vi "aoc-2025-d01-2.vi"() -> ()   [LabVIEW 2020]
uses:
  <vilib>/Utility/miscctls.llb/LVRowAndColumnTypeDef.ctl
panel:
  out "min value":i32
  out "max value":i32
  out "Table Control":string[][](table)
  out "answer":i32
  out "input":i32[](array[numeric])
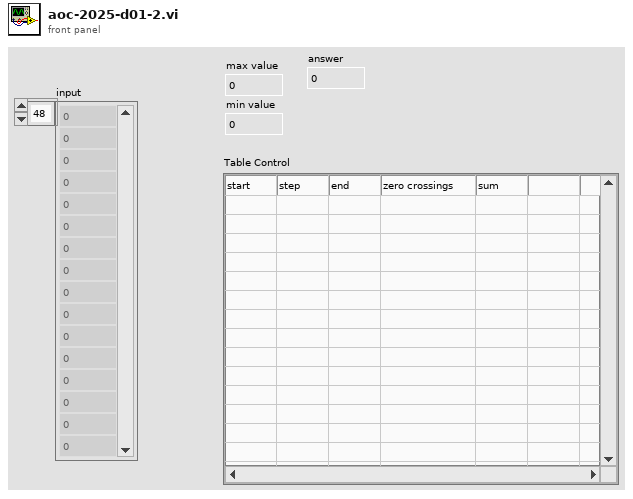
[diagram p1: front panel]
types:
  T1 = typedef "LVRowAndColumnTypeDef.ctl" = cluster{"Row":i32, "Column":i32}
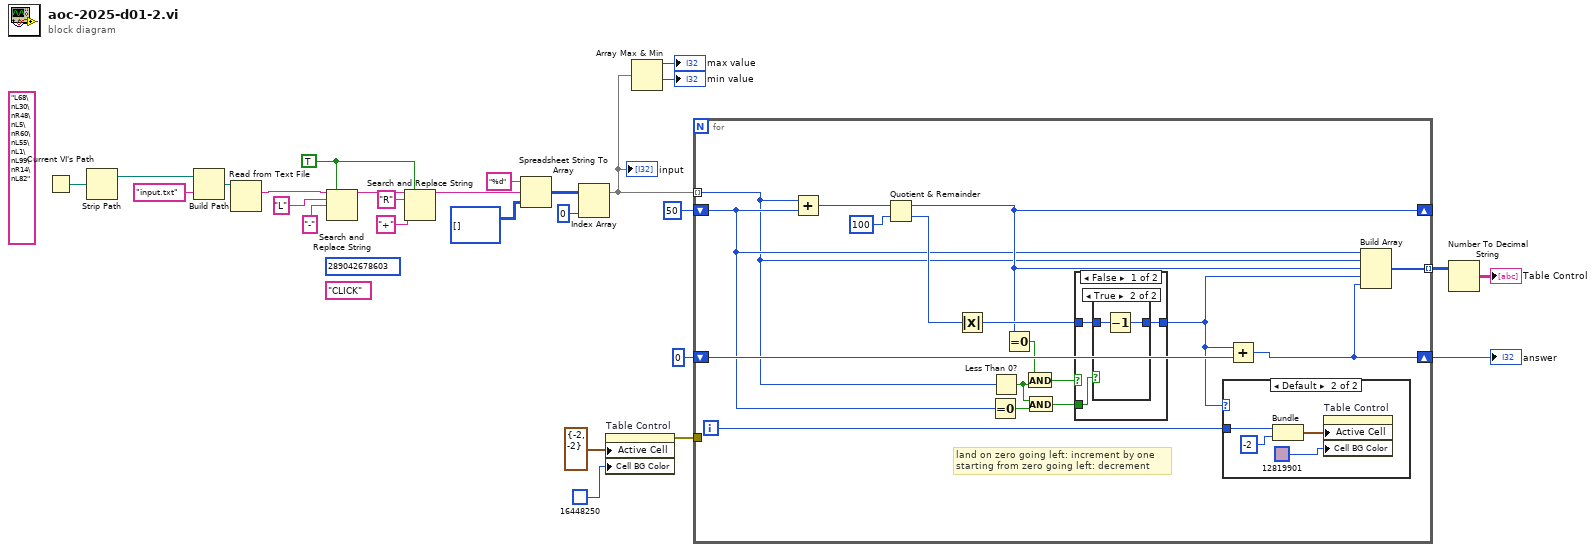
[diagram p0: block diagram]
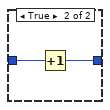
[diagram p3: hidden frame]
diagram:
  (unwired) "CLICK"
  (unwired) u64 289042678603
  (unwired) "L68\nL30\nR48\nL5\nR60\nL55\nL1\nL99\nR14\nL82"
  w26 = TRUE ("replace all? (F)")
  n1 = Current VI's Path() -> (path=w17:path)
  n2 = Strip Path(path=w17) -> (stripped path=w16:path)  [unwired: 1 out]
  n3 = Build Path(base path=w16, name or relative path="input.txt") -> (appended path=w14:path)
  n4 = Read from Text File(file (use dialog)=w14) -> (text=w8:string)  [unwired: 3 in, 3 out]
  n5 = Search and Replace String(replace all?=w26, input string=w8, search string="L" ("replace string (\"\")"), replace string="-" ("replace string (\"\")")) -> (result string=w27:string)  [unwired: 4 in, 3 out]
  n6 = Search and Replace String(replace all?=w26, input string=w27, search string="R", replace string="+" ("replace string (\"\")")) -> (result string=w9:string)  [unwired: 4 in, 3 out]
  n7 = Spreadsheet String To Array(format string="%d", spreadsheet string=w9, array type (2D Dbl)=i32[][] []) -> (array=w7:i32[][])  [unwired: 1 in]
  n8 = Index Array(array=w7, index (col)=0 ("disabled index (col)")) -> (element=w6:i32[])  [unwired: 1 in]
  "input" <- w6
  n9 = property on="Table Control" class="Tbl (strict)"("Active Cell"=T1 {"Row"=-2, "Column"=-2} ("Active Cell:Active Cell"), "Cell BG Color"=u32 16448250 ("Active Cell:Cell Background Color")) -> (error out=w3:errorcluster)  [unwired: 2 in, 1 out]
  n10 = Array Max & Min(array=w6) -> (max value=→"max value":i32, min value=→"min value":i32)  [unwired: 2 out]
  n11 = for {
    tunnel: w6 -> [w28] mode=indexing
    shift-right: [w34] -> _
    shift-left: 50 -> [w32]
    shift-right: [w42] -> w12
    shift-left: 0 -> [w43]
    tunnel: [w41] -> w11 mode=indexing
    tunnel: w3 -> [_]
    i -> [w39]
    # "land on zero going left: increment by one\nstarting from zero going left: decrement"
    n12 = Add(x=w28, y=w32) -> (x+y=w40:i32)
    n13 = Quotient & Remainder(x=w40, y=100) -> (x-y*floor(x/y)=w34:i32, floor(x/y)=w37:i32)
    n14 = Absolute Value(x=w37) -> (abs(x)=w38:i32)
    n15 = Equal To 0?(x=w32) -> (x = 0?=w31:bool)
    n16 = Less Than 0?(x=w28) -> (x < 0?=w29:bool)
    n17 = Equal To 0?(x=w34) -> (x = 0?=w33:bool)
    n18 = And(x=w33, y=w29) -> (x .and. y?=w35:bool)
    n19 = And(x=w29, y=w31) -> (x .and. y?=w30:bool)
    n20 = case shown="False" w35 {
      tunnel: w38 -> [w47 w52]
      tunnel: [w46 w51] -> w36
      tunnel: w30 -> [w45 _]
      frame False {
        n21 = case shown="True" w45 {
          tunnel: w47 -> [w48 w50]
          tunnel: [w48 w49] -> w46
          frame False {
          }
          frame True {
            n22 = Decrement(x=w50) -> (x-1=w49:i32)
          }
        }
      }
      frame True {
        n23 = Increment(x=w52) -> (x+1=w51:i32)
      }
    }
    n24 = case shown="Default" w36 {
      tunnel: w39 -> [_ w55]
      frame 0 {
      }
      frame Default {
        n25 = Bundle(w55, -2) -> (w53:cluster{i32, i32})  [unwired: 1 in]
        n26 = property on="Table Control" class="Tbl (strict)"("Active Cell"=w53, "Cell BG Color"=u32 12819901 ("Active Cell:Cell Background Color")) -> ()  [unwired: 2 in, 2 out]
      }
    }
    n27 = Add(x=w36, y=w43) -> (x+y=w42:i32)
    n28 = Build Array(w32, w28, w34, w36, w42) -> (w41:i32[])
  }
  "answer" <- w12
  n29 = Number To Decimal String(number=w11) -> (decimal integer string=→"Table Control":string[][])  [unwired: 1 in]
